vi "字符串案例之字符串公式解析(上).vi"() -> ()   [LabVIEW 2018]
panel:
  out "数组 2":string[](array[string])
  out "数组":dbl[](array[numeric])
  in  "字符串":string
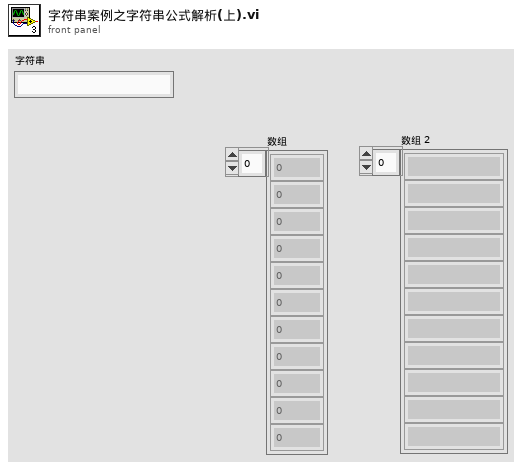
[diagram p1: front panel]
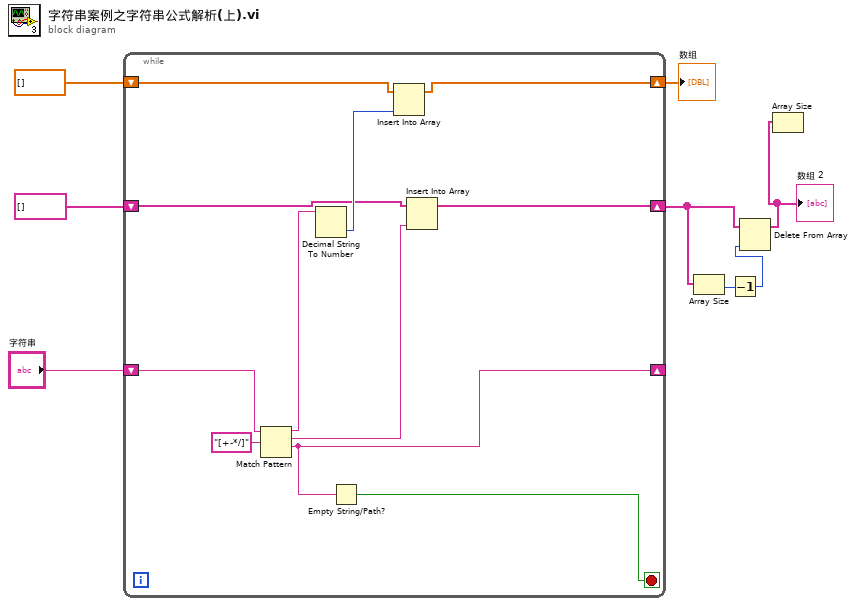
[diagram p0: block diagram]
diagram:
  n1 = while {
    shift-right: [w14] -> w1
    shift-left: dbl[] [] -> [w15]
    shift-right: [w11] -> w5
    shift-left: string[] [] -> [w12]
    shift-right: [w10] -> _
    shift-left: "字符串" -> [w18]
    stop <- w9 stop-if-true
    n2 = Match Pattern(string=w18, regular expression="[+-*/]" ("正则表达式")) -> (before substring=w17:string, match substring=w13:string, after substring=w10:string)  [unwired: 1 in, 1 out]
    n3 = Decimal String To Number(string=w17) -> (number=w16:i32)  [unwired: 2 in, 1 out]
    n4 = Empty String/Path?(string/path=w10) -> (empty?=w9:bool)
    n5 = Insert Into Array(array=w15, new element=w16) -> (w14:dbl[])  [unwired: 1 in]
    n6 = Insert Into Array(array=w12, new element=w13) -> (w11:string[])  [unwired: 1 in]
  }
  "数组" <- w1
  n7 = Array Size(array=w5) -> (size(s)=w4:i32)
  n8 = Decrement(x=w4) -> (x-1=w3:i32)
  n9 = Delete From Array(array=w5, index=w3) -> (array with subset deleted=w2:string[])  [unwired: 1 in, 1 out]
  "数组 2" <- w2
  n10 = Array Size(array=w2) -> ()  [unwired: 1 out]
